vi "Initialize Global Stop.vi"(8 "error in (no error)":errorcluster) -> (0 "error out":errorcluster {"code" min=0 max=0}, 3 "Stop Ref":T1)   [LabVIEW 2015, in "J1939 Addon Engine.lvlib" / "Stop FG.lvlib"]
uses:
  Stop FG.lvlib
  Stop Global Ref.ctl
  Stop Global Commands.ctl
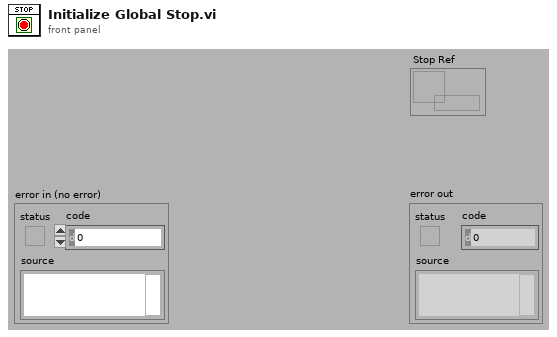
[diagram p1: front panel]
types:
  T1 = typedef "J1939 Addon Engine.lvlib/Stop FG.lvlib/Stop Global Ref.ctl" = refnum<data-value>
  T2 = typedef "J1939 Addon Engine.lvlib/Stop FG.lvlib/Stop Global Commands.ctl" = enum16{"Write", "Read", "Reset"}
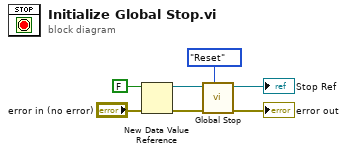
[diagram p0: block diagram]
diagram:
  n1 = New Data Value Reference(data value=FALSE, error in="error in (no error)") -> (data value reference=w5:refnum<data-value>, error out=w4:errorcluster)
  n2 = call "Global Stop.vi"("Command"=Stop_Global_Commands."Reset", "error in (no error)"=w4, "Stop Ref"=w5) -> ("error out"=→"error out":errorcluster, "Stop Ref out"=→"Stop Ref":T1)  [unwired: 6 in, 1 out]
